vi "furmula_distance_conversion_vi.vi"(1 "Schieberegler":dbl) -> (0 "Numeric":dbl)   [LabVIEW 2020]
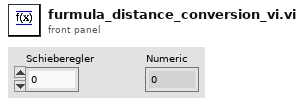
[diagram p1: front panel]
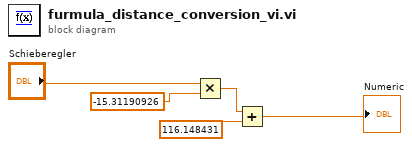
[diagram p0: block diagram]
diagram:
  n1 = Multiply(x="Schieberegler", y=-15.31190926) -> (x*y=w2:dbl)
  n2 = Add(x=w2, y=116.148431) -> (x+y=→"Numeric":dbl)
